vi "Generate Linear Accel Segment.vi"(6 "Index":i32, 9 "Linear Info":T2, 11 "Speeds":T1={"maxV (fps)"=20.0, "Accel Limit (fps^2)"=20.0, "Initial V (fps)"=0.0, "Sample Period (s)"=0.02, "Jerk Limit (fps^3)"=0.0, "Front Distances"={"distance (ft)"=0.0, "baseline (ft)"=0.0, "high (ft)"=0.0}, "Back Distances"={"distance (ft)"=0.0, "baseline (ft)"=0.0, "high (ft)"=0.0}}) -> (0 "Valid":bool, 1 "Final Position":cluster{dbl, dbl, dbl}, 2 "Trajectory Segment":T3, 3 "Speeds Out":T1={"maxV (fps)"=0.0, "Accel Limit (fps^2)"=0.0, "Initial V (fps)"=0.0, "Sample Period (s)"=0.02, "Jerk Limit (fps^3)"=0.0, "Front Distances"={"distance (ft)"=0.0, "baseline (ft)"=0.0, "high (ft)"=0.0}, "Back Distances"={"distance (ft)"=0.0, "baseline (ft)"=0.0, "high (ft)"=0.0}})   [LabVIEW 2018]
panel:
  out "Waveform Graph":dbl[][](graph)
  out "XY Graph":cluster{dbl, dbl}[](graph)
  out "Segment Time (s)":dbl
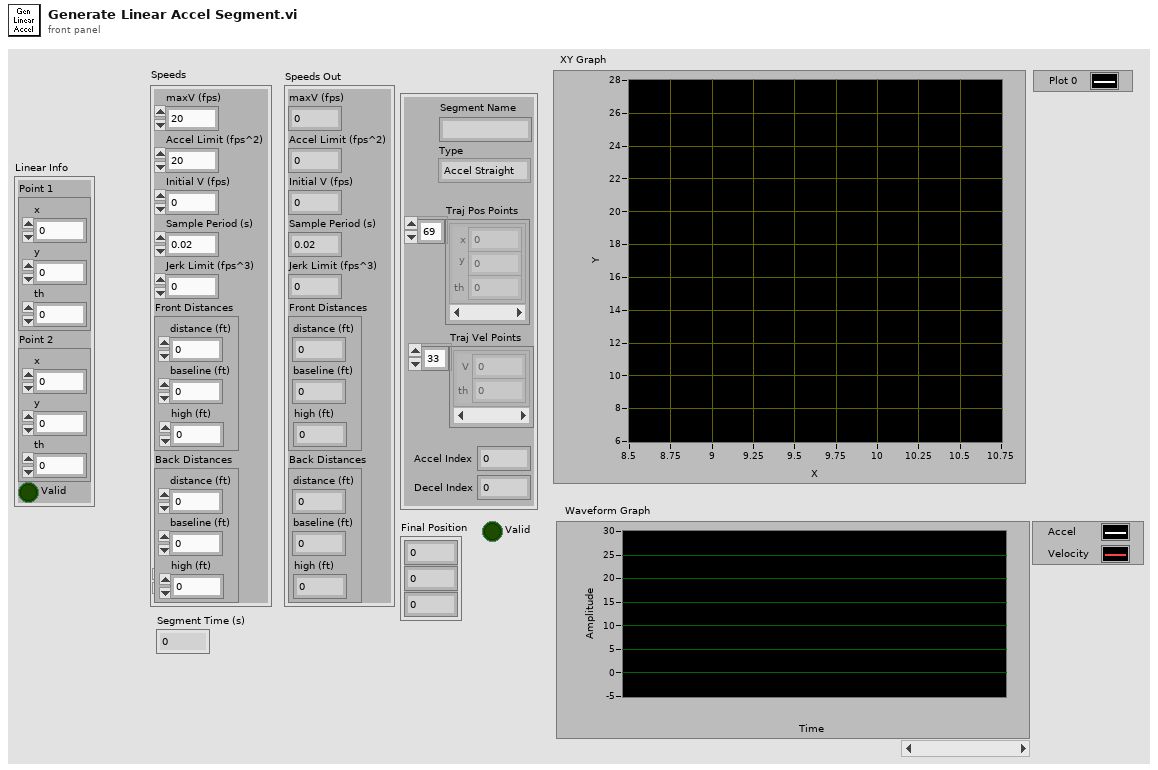
[diagram p1: front panel]
types:
  T1 = cluster{"maxV (fps)":dbl, "Accel Limit (fps^2)":dbl, "Initial V (fps)":dbl, "Sample Period (s)":dbl, "Jerk Limit (fps^3)":dbl, "Front Distances":cluster{"distance (ft)":dbl, "baseline (ft)":dbl, "high (ft)":dbl}, "Back Distances":cluster{"distance (ft)":dbl, "baseline (ft)":dbl, "high (ft)":dbl}}
  T2 = cluster{"Point 1":cluster{"x":dbl, "y":dbl, "th":dbl}, "Point 2":cluster{"x":dbl, "y":dbl, "th":dbl}, "Valid":bool}
  T3 = cluster{"Segment Name":string, "Type":enum16{"Accel Straight", "Const Straight", "Blend", "Circle"}, "Traj Pos Points":cluster{"x":dbl, "y":dbl, "th":dbl}[], "Traj Vel Points":cluster{"V":dbl, "th":dbl}[], "Accel Index":i32, "Decel Index":i32}
  T4 = enum16{"Accel Straight", "Const Straight", "Blend", "Circle"}
  T5 = cluster{"distance (ft)":dbl, "baseline (ft)":dbl, "high (ft)":dbl}
  T6 = cluster{string, "Type":enum16{"Accel Straight", "Const Straight", "Blend", "Circle"}, cluster{dbl, dbl, dbl}[], cluster{"velocity":dbl, dbl}[], "Accel Index":i32, "Decel Index":i32}
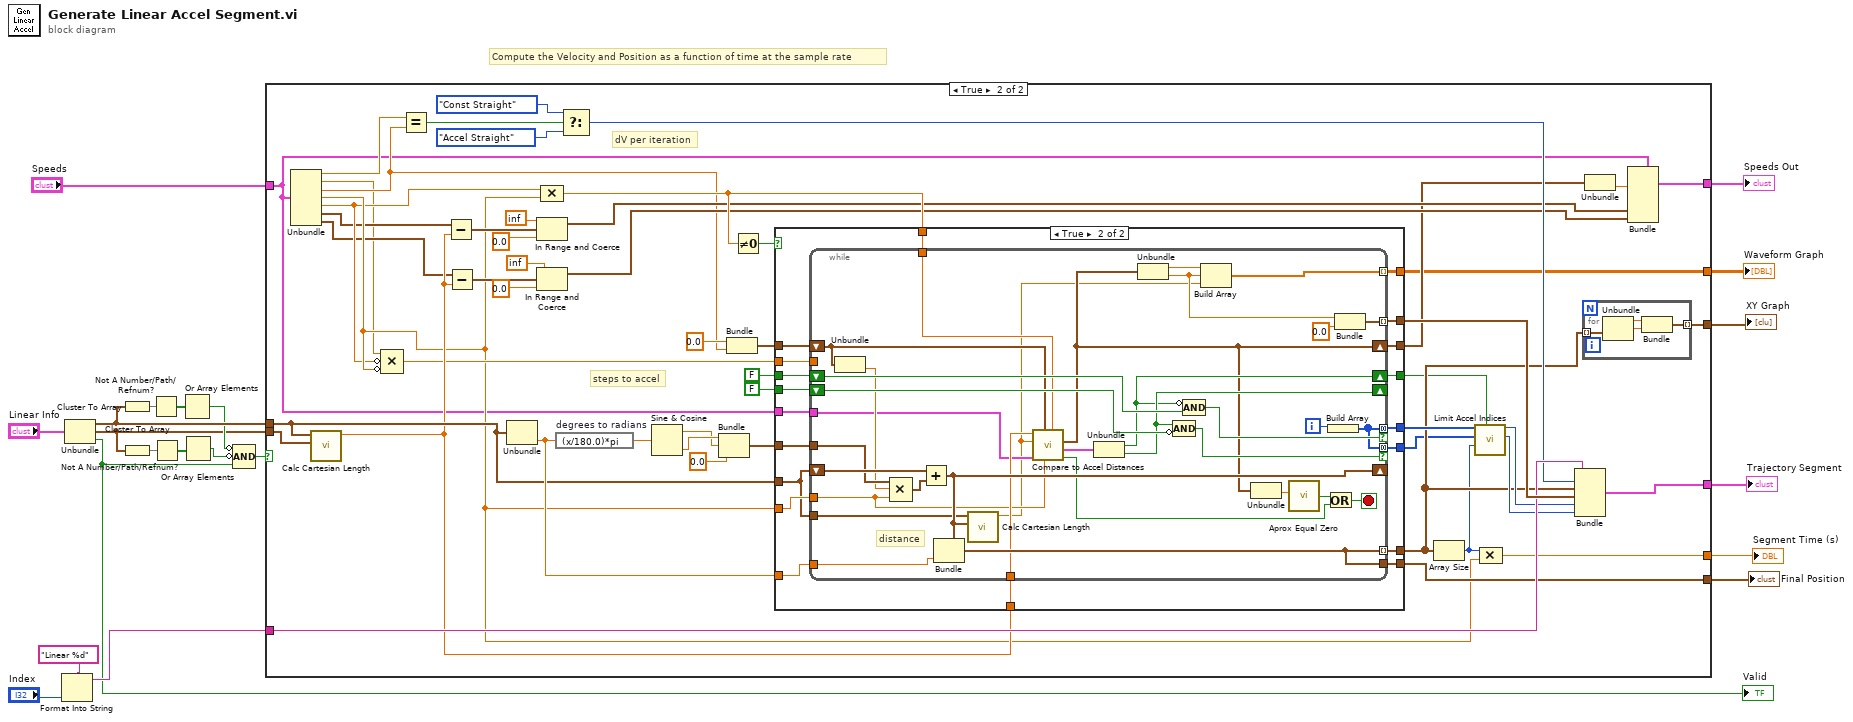
[diagram p0: block diagram]
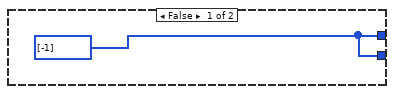
[diagram p3: hidden frame]
diagram:
  # "Compute the Velocity and Position as a function of time at the sample rate"
  n1 = Format Into String(format string="Linear %d", "Index") -> (resulting string=w13:string)  [unwired: 2 in, 1 out]
  n2 = Unbundle("Linear Info") -> ("Point 1"=w9:cluster{"x":dbl, "y":dbl, "th":dbl}, "Point 2"=w4:cluster{"x":dbl, "y":dbl, "th":dbl}, "Valid"=w10:bool)
  "Valid" <- w10
  n3 = Cluster To Array(cluster=w9) -> (array=w8:dbl[])
  n4 = Cluster To Array(cluster=w4) -> (array=w5:dbl[])
  n5 = Not A Number/Path/Refnum?(number/path/refnum=w8) -> (NaN/Path/Refnum?=w7:bool[])
  n6 = Not A Number/Path/Refnum?(number/path/refnum=w5) -> (NaN/Path/Refnum?=w3:bool[])
  n7 = Or Array Elements(Boolean array=w7) -> (logical OR=w6:bool)
  n8 = Or Array Elements(Boolean array=w3) -> (logical OR=w2:bool)
  n9 = Compound Arithmetic op=AND(invert w6, invert w2, w10) -> (w11:bool)
  n10 = case shown="True" w11 {
    tunnel: [_ w76] -> w21
    tunnel: w13 -> [_ w70]
    tunnel: [_ w66] -> w20
    tunnel: [w22 w65] -> w19
    tunnel: [_ w62] -> w18
    tunnel: "Speeds" -> [w23 w24]
    tunnel: [w23 w61] -> w16
    tunnel: w9 -> [w22 w55]
    tunnel: w4 -> [_ w58]
    tunnel: [_ w25] -> w1
    frame False {
    }
    frame True {
      # "steps to accel"
      # "dV per iteration"
      n11 = Unbundle(w24) -> ("maxV (fps)"=w60:dbl, "Accel Limit (fps^2)"=w26:dbl, "Initial V (fps)"=w30:dbl, "Sample Period (s)"=w38:dbl, "Jerk Limit (fps^3)"=w36:dbl, "Front Distances"=w35:T5, "Back Distances"=w32:T5)
      n12 = call "Calc Cartesian Length.vi"("Point 2"=w58, "Point 1"=w55) -> ("Length (f)"=w46:dbl)  [unwired: 8 in, 1 out]
      n13 = Compound Arithmetic op=MULTIPLY(w26, invert w36, invert w38) -> (w39:dbl)
      n14 = Equal?(x=w60, y=w30) -> (x = y?=w59:bool)
      n15 = Subtract(x=w35, y=w46) -> (x-y=w51:T5)
      n16 = Subtract(x=w32, y=w46) -> (x-y=w45:T5)
      n17 = Unbundle(w55) -> ("th"=w64:dbl)  [unwired: 2 out]
      n18 = In Range and Coerce(upper limit=inf, x=w51, lower limit=0.0) -> (coerced(x)=w34:T5)  [unwired: 1 out]
      n19 = In Range and Coerce(upper limit=inf, x=w45, lower limit=0.0) -> (coerced(x)=w33:T5)  [unwired: 1 out]
      n20 = Compound Arithmetic op=MULTIPLY(w36, w38) -> (w57:dbl)
      n21 = expression code="(x/180.0)*pi" "degrees to radians"(w64) -> (w63:dbl)
      n22 = Select(t=T4."Const Straight" ("Type"), s=w59, f=T4."Accel Straight" ("Type")) -> (s? t:f=w67:T4)
      n23 = Sine & Cosine(0:w63) -> (1:w71:dbl, 2:w72:dbl)
      n24 = Bundle(w72, w71, 0.0) -> (w74:cluster{dbl, dbl, dbl})  [unwired: 1 in]
      n25 = Bundle(0.0, "Initial V (fps)"=w30) -> (w29:cluster{dbl, "Initial V (fps)":dbl})  [unwired: 1 in]
      n26 = Not Equal To 0?(x=w57) -> (x != 0?=w56:bool)
      n27 = case shown="True" w56 {
        tunnel: [_ w100] -> w75
        tunnel: w74 -> [_ w99]
        tunnel: [_ w98] -> w65
        tunnel: w64 -> [_ w97]
        tunnel: [_ w96] -> w43
        tunnel: [_ w95] -> w28
        tunnel: w57 -> [_ w94]
        tunnel: w38 -> [_ w93]
        tunnel: w55 -> [_ w92]
        tunnel: w46 -> [_ w91]
        tunnel: FALSE -> [_ w90]
        tunnel: [w81 w89] -> w49
        tunnel: w24 -> [_ w88]
        tunnel: FALSE -> [_ w87]
        tunnel: [w81 w86] -> w42
        tunnel: [_ w85] -> w40
        tunnel: w39 -> [_ w84]
        tunnel: w29 -> [_ w83]
        tunnel: [_ w82] -> w25
        frame False {
          w81 = i32[] [-1]
        }
        frame True {
          n28 = while {
            tunnel: [w125] -> w96 mode=indexing
            tunnel: w94 -> [w109]
            shift-right: [w102] -> w95
            shift-left: w83 -> [w113]
            tunnel: [w131] -> w100 mode=indexing
            tunnel: w93 -> [w106]
            tunnel: w99 -> [w129]
            tunnel: w97 -> [w132]
            tunnel: [w125] -> w98
            tunnel: w91 -> [w123]
            shift-right: [w127] -> _
            shift-left: w92 -> [w130]
            tunnel: w92 -> [w126]
            shift-right: [w108] -> w85
            shift-left: w90 -> [w122]
            tunnel: [w119] -> w89 mode=concatenating if=w121
            tunnel: w88 -> [w105]
            shift-right: [w111] -> _
            shift-left: w87 -> [w120]
            tunnel: [w119] -> w86 mode=concatenating if=w118
            tunnel: w84 -> [_]
            tunnel: [w107] -> w82 mode=indexing
            i -> [w124]
            stop <- w116 stop-if-true
            # "distance"
            n29 = Unbundle(w113) -> ("Initial V (fps)"=w114:dbl)  [unwired: 1 out]
            n30 = Compound Arithmetic op=MULTIPLY(w129, w114, w106) -> (w128:cluster{dbl, dbl, dbl})
            n31 = Add(x=w130, y=w128) -> (x+y=w127:cluster{dbl, dbl, dbl})
            n32 = Bundle(cluster=w127, w132) -> (w125:cluster{dbl, dbl, dbl})  [unwired: 2 in]
            n33 = call "Calc Cartesian Length.vi"("Point 2"=w127, "Point 1"=w126) -> ("Length (f)"=w101:dbl)  [unwired: 8 in, 1 out]
            n34 = call "Compare to Accel Distances.vi"("dA"=w109, "Sample Period (s)"=w106, "Values"=w113, "Speeds"=w105, "Current  Length"=w101, "Total Segment Length"=w123) -> ("End Loop"=w117:bool, "Ends"=w112:cluster{"Accel End":bool, "Decel End":bool}, "Values out"=w102:cluster{"accel":dbl, "velocity":dbl})  [unwired: 2 in, 1 out]
            n35 = Unbundle(w112) -> ("Accel End"=w108:bool, "Decel End"=w111:bool)
            n36 = Unbundle(w102) -> ("accel"=w103:dbl, "velocity"=w104:dbl)
            n37 = Compound Arithmetic op=AND(w111, invert w120) -> (w118:bool)
            n38 = Compound Arithmetic op=AND(invert w108, w122) -> (w121:bool)
            n39 = Build Array(w103, w104, w101) -> (w107:dbl[])
            n40 = Unbundle(w102) -> ("velocity"=w110:dbl)  [unwired: 1 out]
            n41 = call "Aprox Equal Zero.vi"("maxV (fps)"=w110) -> ("Boolean"=w115:bool)  [unwired: 10 in]
            n42 = Or(x=w115, y=w117) -> (x .or. y?=w116:bool)
            n43 = Build Array(w124) -> (w119:i32[])
            n44 = Bundle("velocity"=w104, 0.0) -> (w131:cluster{"velocity":dbl, dbl})  [unwired: 1 in]
          }
        }
      }
      n45 = Array Size(array=w43) -> (size(s)=w41:i32)
      n46 = call "Limit Accel Indices.vi"("Last Accel"=w40, "Size"=w41, "Decel"=w42, "Accel"=w49) -> ("Decel Index"=w48:i32, "Accel Index"=w50:i32)  [unwired: 6 in]
      n47 = Compound Arithmetic op=MULTIPLY(w41, w38) -> (w66:dbl)
      n48 = Bundle(w70, "Type"=w67, w43, w75, "Accel Index"=w50, "Decel Index"=w48) -> (w76:T6)  [unwired: 1 in]
      n49 = for {
        tunnel: w43 -> [w80] mode=indexing
        tunnel: [w77] -> w62 mode=indexing
        n50 = Unbundle(w80) -> (w79:dbl, w78:dbl)  [unwired: 1 out]
        n51 = Bundle(w79, w78) -> (w77:cluster{dbl, dbl})  [unwired: 1 in]
      }
      n52 = Unbundle(w28) -> ("Initial V (fps)"=w27:dbl)  [unwired: 1 out]
      n53 = Bundle(cluster=w24, "Initial V (fps)"=w27, "Front Distances"=w34, "Back Distances"=w33) -> (w61:T1)  [unwired: 4 in]
    }
  }
  "Trajectory Segment" <- w21
  "Segment Time (s)" <- w20
  "Final Position" <- w19
  "XY Graph" <- w18
  "Speeds Out" <- w16
  "Waveform Graph" <- w1
